vi "AlliGator Create Cursors for Square Gated IRF Fit.vi"(8 "Error In":errorcluster, 11 "Decay Graph":refnum<vi>) -> (0 "Error Out":errorcluster, 3 "# Added Cursors":i32)   [LabVIEW 2021, in "AlliGator Decay Analysis.lvlib" / "AlliGator IRF.lvlib"]
doc: "Creates 5 cursors (tr1, tr2, tf1, tf2 and ten) used to define the different transitions between domains in a square gate."
uses:
  AlliGator IRF.lvlib
  <vilib>/Utility/miscctls.llb/LVCursorListTypeDef.ctl
  Graphs/XY Graph/XY Graph Add-Ons.lvlib
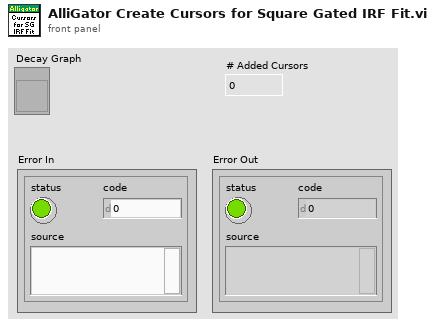
[diagram p1: front panel]
types:
  T1 = typedef "LVCursorListTypeDef.ctl" = cluster{"Name":string, "Color":u32, "Style":u8, "Point Style":u8, "Name Visible":bool, "Allow Drag":bool, "Cursor Mode":u32, "Plot":i32, "Index":i32, "Position":cluster{"X":dbl, "Y":dbl}, "X Scale":u32, "Y Scale":u32, "Watch Plots":i32[], "Watch All Plots":bool, "Plot Area":i32, "Label Offset":cluster{"X":dbl, "Y":dbl}}[]
  T2 = cluster{"Name":string, "Color":u32, "Style":u8, "Point Style":u8, "Name Visible":bool, "Allow Drag":bool, "Cursor Mode":u32, "Plot":i32, "Index":i32, "Position":cluster{"X":dbl, "Y":dbl}, "X Scale":u32, "Y Scale":u32, "Watch Plots":i32[], "Watch All Plots":bool, "Plot Area":i32, "Label Offset":cluster{"X":dbl, "Y":dbl}}
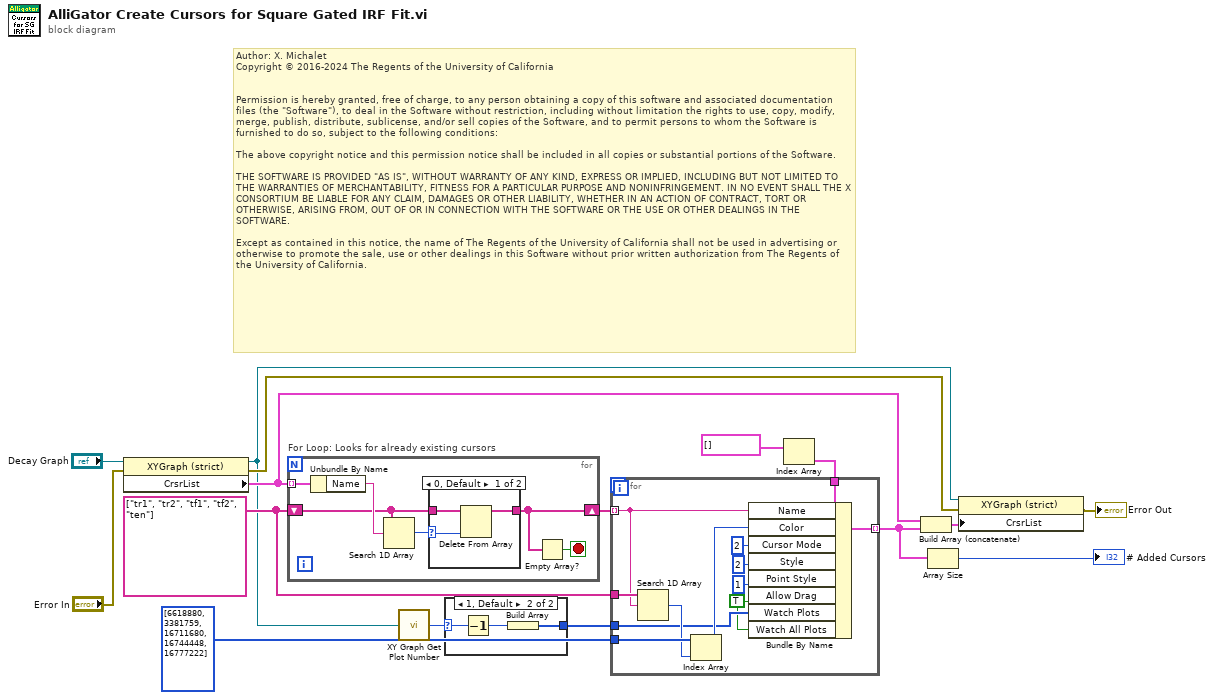
[diagram p0: block diagram]
diagram:
  w13 = string[] ["tr1", "tr2", "tf1", "tf2", "ten"]
  # "Author: X. Michalet\nCopyright © 2016-2024 The Regents of the University of California\n \n\nPermission is hereby granted, free of charge, to any person obtaining a copy of this software and associated documentation files (the \"Software\"), to deal in the Software without restriction, including without limitation the rights to use, copy, modify, merge, publish, distribute, sublicense, and/or sell copies of the Software, and to permit persons to whom the Software is furnished to do so, subject to the following conditions:\n\nThe above copyright notice and this permission notice shall be included in all copies or substantial portions of the Software.\n\nTHE SOFTWARE IS PROVIDED \"AS IS\", WITHOUT WARRANTY OF ANY KIND, EXPRESS OR IMPLIED, INCLUDING BUT NOT LIMITED TO THE WARRANTIES OF MERCHANTABILITY, FITNESS FOR A PARTICULAR PURPOSE AND NONINFRINGEMENT. IN NO EVENT SHALL THE X CONSORTIUM BE LIABLE FOR ANY CLAIM, DAMAGES OR OTHER LIABILITY, WHETHER IN AN ACTION OF CONTRACT, TORT OR OTHERWISE, ARISING FROM, OUT OF OR IN CONNECTION WITH THE SOFTWARE OR THE USE OR OTHER DEALINGS IN THE SOFTWARE.\n\nExcept as contained in this notice, the name of The Regents of the University of California shall not be used in advertising or otherwise to promote the sale, use or other dealings in this Software without prior written authorization from The Regents of the University of California."
  n1 = property class="XYGraph (strict)"(reference="Decay Graph", error in="Error In") -> (reference out=w3:refnum<vi>, error out=w7:errorcluster, "CrsrList"=w9:T1)
  n2 = for "For Loop: Looks for already existing cursors" {
    tunnel: w9 -> [w22] mode=indexing
    shift-right: [w18] -> w14
    shift-left: w13 -> [w19]
    stop <- w17 stop-if-true
    n3 = Unbundle By Name(w22) -> ("Name"=w21:string)
    n4 = Search 1D Array(1D array=w19, element=w21) -> (index of element=w20:i32)  [unwired: 1 in]
    n5 = case shown="0, Default" w20 {
      selector: w20 -> [w24 _]
      tunnel: w19 -> [w25 w26]
      tunnel: [w23 w26] -> w18
      frame 0, Default {
        n6 = Delete From Array(array=w25, index=w24) -> (array with subset deleted=w23:string[])  [unwired: 1 in, 1 out]
      }
      frame -1 {
      }
    }
    n7 = Empty Array?(array=w18) -> (empty?=w17:bool)
  }
  n8 = call "XY Graph Get Plot Number.vi"("XYGraph"=w3) -> ("# Plots"=w2:i32)  [unwired: 8 in]
  n9 = case shown="1, Default" w2 {
    selector: w2 -> [_ w29]
    tunnel: [_ w27] -> w1
    frame 0 {
    }
    frame 1, Default {
      n10 = Decrement(x=w29) -> (x-1=w28:i32)
      n11 = Build Array(w28) -> (w27:i32[])
    }
  }
  n12 = Index Array(array=T1 [] ("Cursor List")) -> (element=w10:T2)  [unwired: 1 in]
  n13 = for {
    tunnel: w14 -> [w38] mode=indexing
    tunnel: w13 -> [w41]
    tunnel: u32[] [6618880, 3381759, 16711680, 16744448, 16777222] -> [w40]
    tunnel: w10 -> [w37]
    tunnel: [w34] -> w5 mode=indexing
    tunnel: w1 -> [w31]
    w30 = TRUE ("Allow Drag")
    n14 = Search 1D Array(1D array=w41, element=w38) -> (index of element=w39:i32)  [unwired: 1 in]
    n15 = Index Array(array=w40, index=w39) -> (element=w36:u32)
    n16 = Bundle By Name(cluster=w37, "Name"=w38, "Color"=w36, "Cursor Mode"=u32 2, "Style"=u8 2, "Point Style"=u8 1, "Allow Drag"=w30, "Watch Plots"=w31, "Watch All Plots"=w30) -> (w34:T2)
  }
  n17 = Build Array (concatenate)(w9, w5) -> (w8:T1)
  n18 = Array Size(array=w5) -> (size(s)=→"# Added Cursors":i32)
  n19 = property class="XYGraph (strict)"(reference=w3, error in=w7, "CrsrList"=w8) -> (error out=→"Error Out":errorcluster)  [unwired: 1 out]
